vi "Disable Channel.vi"(8 "error in (no error)":errorcluster, 9 "Index":i32, 11 "SigMan in":refnum<class "SignalManager.lvclass">) -> (0 "error out":errorcluster, 3 "SigMan out":refnum<class "SignalManager.lvclass">)   [LabVIEW 2020, in "SignalManager.lvclass"]
uses:
  SignalManager.lvclass
  SignalManager.lvclass/SignalManager.ctl
  Channel/Channel.lvclass
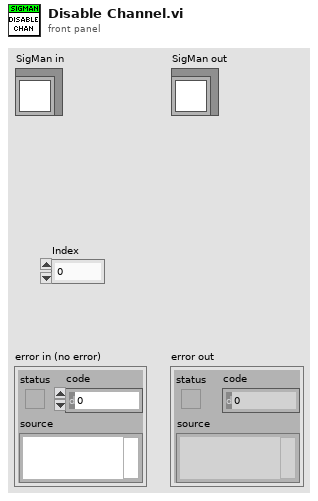
[diagram p1: front panel]
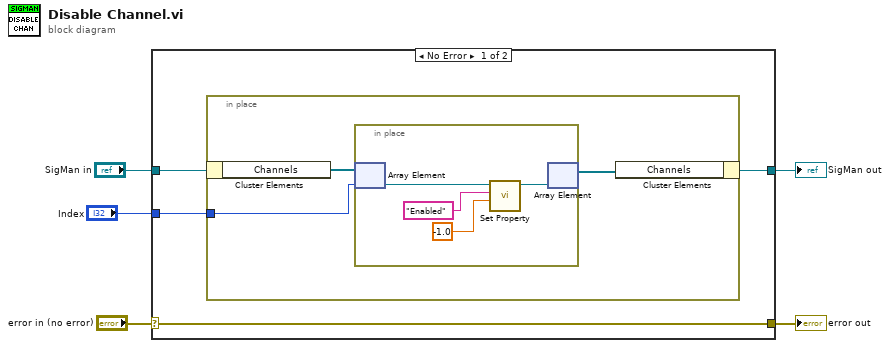
[diagram p0: block diagram]
diagram:
  n1 = case shown="No Error" "error in (no error)" {
    selector: "error in (no error)" -> [w9 w18]
    tunnel: [w9 w18] -> w4
    tunnel: [w6 w17] -> w2
    tunnel: "SigMan in" -> [w8 w17]
    tunnel: "Index" -> [w7 _]
    frame No Error {
      n2 = in-place {
        in-place-border: w7 -> [w11]
        n3 = in-place-cluster #1(w8) -> ("Channels"=w12:refnum<class "Channel.lvclass">[])
        n4 = in-place {
          n5 = in-place-array #2(w12, w11) -> (w15:refnum<class "Channel.lvclass">)
          n6 = call "Set Property.vi"("Value"=-1.0, "Property"="Enabled", "Channel in"=w15) -> ("Channel out"=w13:refnum<class "Channel.lvclass">)  [unwired: 7 in, 1 out]
          n7 = in-place-array #2(w13) -> (w10:refnum<class "Channel.lvclass">[])  [unwired: 1 out]
        }
        n8 = in-place-cluster #1("Channels"=w10) -> (w6:refnum<class "SignalManager.lvclass">)
      }
    }
    frame Error {
    }
  }
  "error out" <- w4
  "SigMan out" <- w2
